vi "get last index.vi"(11 "Channel":T1={"Name"="", "Modbus Type"=enum."Coil", "Veristand Type"=enum."Output", "Mapping"={"DataType"=enum."Double", "Starting Address"=0, "Sub-Index (Bool)"=0, "VS Reference"=0}}) -> (3 "Last Index":u16)   [LabVIEW 2020, in "Modbus Master System Explorer.lvlib"]
uses:
  System Explorer/Modbus Master System Explorer.lvlib
  Shared/Controls/Data Model/Channel.ctl
  System Explorer/SubVIs/Modbus Type.ctl
  <vilib>/NI VeriStand/Custom Device API/Custom Device Channel Type.ctl
  Shared/Controls/Data Model/Mapping.ctl
  Shared/Controls/Data Model/DataType.ctl
  <vilib>/NI VeriStand/Custom Device API/Custom Device Item Ref.ctl
  Shared/Modbus Master Shared.lvlib
  <vilib>/NI VeriStand/Custom Device API/Custom Device API.lvlib
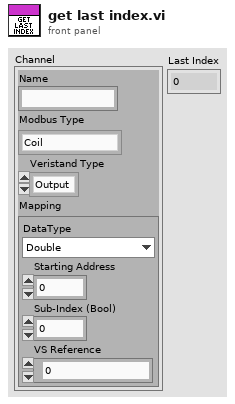
[diagram p1: front panel]
types:
  T1 = typedef "Modbus Master Shared.lvlib/Channel.ctl" = cluster{"Name":string, "Modbus Type":T2, "Veristand Type":T3, "Mapping":T4}
  T2 = typedef "Modbus Master Shared.lvlib/Modbus Type.ctl" = enum16{"Coil", "Discrete Input", "Holding Register", "Input Register"}
  T3 = typedef "Custom Device API.lvlib/Custom Device Channel Type.ctl" = enum16{"Input", "Output"}
  T4 = typedef "Modbus Master Shared.lvlib/Mapping.ctl" = cluster{"DataType":T5, "Starting Address":u16, "Sub-Index (Bool)":u16, "VS Reference":T6}
  T5 = typedef "Modbus Master Shared.lvlib/DataType.ctl" = enum16{"Double", "Single", "I64", "I32", "I16", "I8", "U64", "U32", "U16", "U8", "Boolean"}
  T6 = typedef "Custom Device API.lvlib/Custom Device Item Ref.ctl" = u64
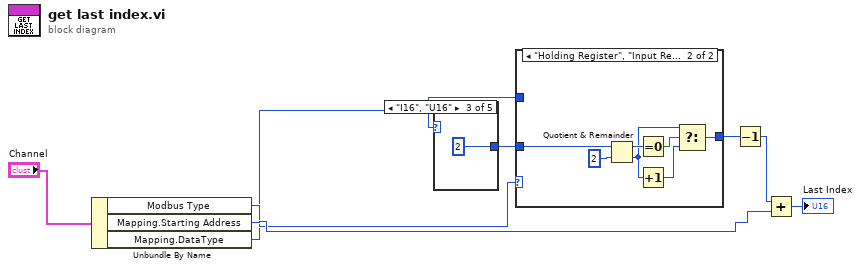
[diagram p0: block diagram]
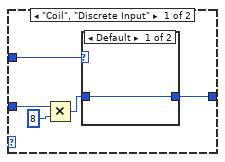
[diagram p2: hidden frame]
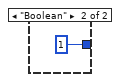
[diagram p3: hidden frame]
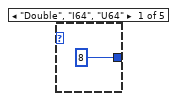
[diagram p4: hidden frame]
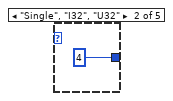
[diagram p5: hidden frame]
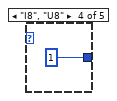
[diagram p6: hidden frame]
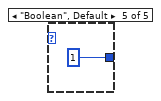
[diagram p7: hidden frame]
diagram:
  n1 = Unbundle By Name("Channel") -> ("Modbus Type"=w7:T2, "Mapping.Starting Address"=w8:u16, "Mapping.DataType"=w6:T5)
  n2 = case shown="\"I16\", \"U16\"" w6 {
    tunnel: [u16 8 ("x") u16 4 ("x") u16 2 ("x") u16 1 ("x") u16 1 ("x")] -> w2
    frame "Double", "I64", "U64" {
    }
    frame "Single", "I32", "U32" {
    }
    frame "I16", "U16" {
    }
    frame "I8", "U8" {
    }
    frame "Boolean", Default {
    }
  }
  n3 = case shown="\"Holding Register\", \"Input Register\"" w7 {
    tunnel: w2 -> [w18 w27]
    tunnel: [w15 w21] -> w3
    tunnel: w6 -> [w16 _]
    frame "Coil", "Discrete Input" {
      n4 = Multiply(x=w18, y=u16 8) -> (x*y=w14:u16)
      n5 = case shown="Default" w16 {
        tunnel: [w19 u16 1] -> w15
        tunnel: w14 -> [w19 _]
        frame Default {
        }
        frame "Boolean" {
        }
      }
    }
    frame "Holding Register", "Input Register" {
      n6 = Quotient & Remainder(x=w27, y=u16 2) -> (x-y*floor(x/y)=w25:u16, floor(x/y)=w23:u16)
      n7 = Equal To 0?(x=w25) -> (x = 0?=w24:bool)
      n8 = Increment(x=w23) -> (x+1=w22:u16)
      n9 = Select(t=w23, s=w24, f=w22) -> (s? t:f=w21:u16)
    }
  }
  n10 = Decrement(x=w3) -> (x-1=w4:u16)
  n11 = Add(x=w4, y=w8) -> (x+y=→"Last Index":u16)
